vi "Set Connection DVR.vi"(8 "error in":errorcluster {"code" format="Error %.0f"}, 10 "NATS Connection":refnum<data-value>, 11 "NATS Client in":refnum<class "NATS Client.lvclass">) -> (0 "error out":errorcluster {"code" format="Error %.0f"}, 3 "NATS Client out":refnum<class "NATS Client.lvclass">)   [LabVIEW 2020, in "NATS Client.lvlib" / "NATS Client.lvclass"]
uses:
  NATS Client.lvclass
  NATS Client.lvclass/NATS Client.ctl
  <vilib>/NATS/NATS Core/Controls/nats connection.ctl
  <vilib>/NATS/NATS Core/NATS Core.lvlib
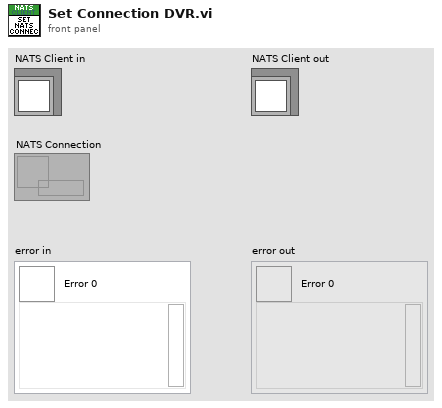
[diagram p1: front panel]
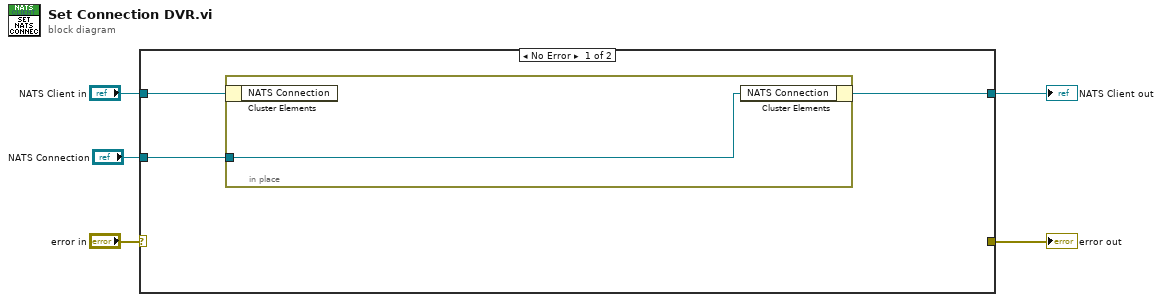
[diagram p0: block diagram]
diagram:
  n1 = case shown="No Error" "error in" {
    selector: "error in" -> [_ w11]
    tunnel: [_ w11] -> w4
    tunnel: [w7 w10] -> w2
    tunnel: "NATS Client in" -> [w8 w10]
    tunnel: "NATS Connection" -> [w6 _]
    frame No Error {
      n2 = in-place {
        in-place-border: w6 -> [w9]
        n3 = in-place-cluster #1(w8) -> ()  [unwired: 1 out]
        n4 = in-place-cluster #1("NATS Connection"=w9) -> (w7:refnum<class "NATS Client.lvclass">)
      }
    }
    frame Error {
    }
  }
  "error out" <- w4
  "NATS Client out" <- w2
